vi "9.vi"() -> ()   [LabVIEW 2023]
uses:
  <vilib>/Utility/file.llb/Write Delimited Spreadsheet (string).vi
panel:
  out "NUME PRENUME":string[](array[string])
  out "note":dbl[][](array[numeric])
  in  "Save Button":bool
  in  "stop":bool
  in  "Array":T1(array[cluster])
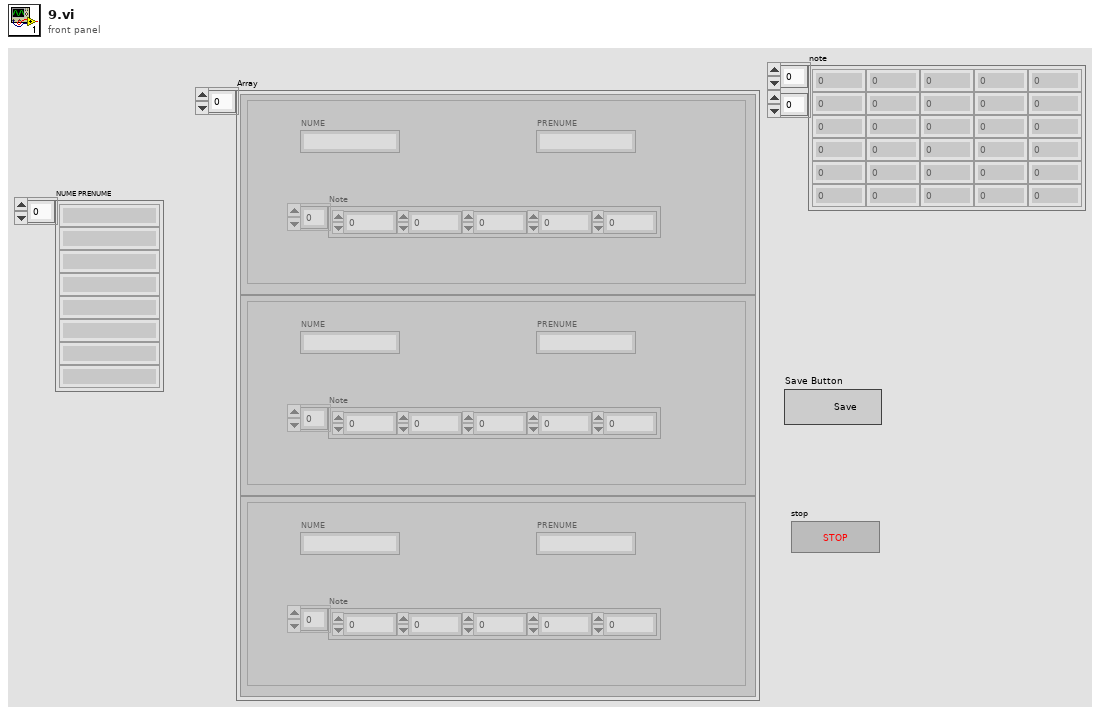
[diagram p1: front panel]
types:
  T1 = cluster{"NUME":string, "PRENUME ":string, "Note":dbl[]}[]
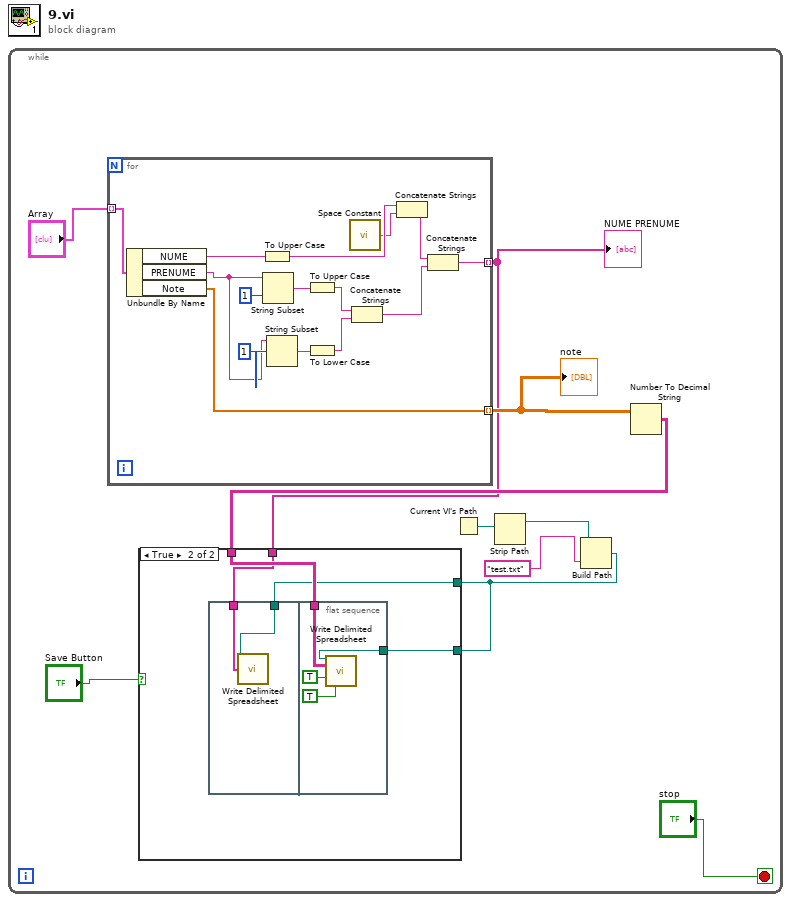
[diagram p0: block diagram]
diagram:
  n1 = while {
    stop <- "stop" stop-if-true
    n2 = for {
      tunnel: "Array" -> [w35] mode=indexing
      tunnel: [w22] -> w2 mode=indexing
      tunnel: [w21] -> w4 mode=indexing
      n3 = Unbundle By Name(w35) -> ("NUME"=w34:string, "PRENUME"=w31:string, "Note"=w21:dbl[])
      n4 = To Upper Case(1:w34) -> (0:w26:string)
      n5 = String Subset(string=w31, length (rest)=1 ("length (rest)")) -> (substring=w30:string)  [unwired: 1 in]
      n6 = String Subset(string=w31, offset (0)=1) -> (substring=w29:string)  [unwired: 1 in]
      n7 = To Upper Case(1:w30) -> (0:w28:string)
      n8 = To Lower Case(string=w29) -> (all lower case string=w27:string)
      n9 = call <vilib>:"Space Constant.vi"() -> ("String"=w25:string)
      n10 = Concatenate Strings(w28, w27) -> (w23:string)
      n11 = Concatenate Strings(w26, w25) -> (w24:string)
      n12 = Concatenate Strings(w24, w23) -> (w22:string)
    }
    "note" <- w4
    "NUME PRENUME" <- w2
    n13 = Current VI's Path() -> (path=w8:path)
    n14 = Strip Path(path=w8) -> (stripped path=w7:path)  [unwired: 1 out]
    n15 = Build Path(base path=w7, name or relative path="test.txt") -> (appended path=w1:path)
    n16 = Number To Decimal String(number=w4) -> (decimal integer string=w3:string[][])  [unwired: 1 in]
    n17 = case shown="True" "Save Button" {
      tunnel: w3 -> [_ w14]
      tunnel: w2 -> [_ w13]
      tunnel: w1 -> [_ w12]
      tunnel: w1 -> [_ w11]
      frame False {
      }
      frame True {
        n18 = flat-sequence {
          tunnel: w13 -> [w16]
          tunnel: w12 -> [w15]
          tunnel: w14 -> [w18]
          tunnel: w11 -> [w17]
          frame #0 {
            n19 = call-poly <vilib>:"Write Delimited Spreadsheet.vi"("file path (dialog if empty)"=w15, "1D data"=w16) -> ()  [unwired: 12 in, 2 out]
          }
          frame #1 {
            n20 = call-poly <vilib>:"Write Delimited Spreadsheet.vi"("file path (dialog if empty)"=w17, "2D data"=w18, "append to file? (new file:F)"=TRUE, "transpose? (no:F)"=TRUE) -> ()  [unwired: 10 in, 2 out]
          }
        }
      }
    }
  }
